vi "FinalizeHWI.vi"(8 "error in (no error)":errorcluster, 10 "Master Device in":refnum<class "Master Device.lvclass">, 11 "Slave_Line in":refnum<class "Slave_Line.lvclass">) -> (0 "error out":errorcluster, 2 "Master Device out":refnum<class "Master Device.lvclass">, 3 "Slave_Line out":refnum<class "Slave_Line.lvclass">)   [LabVIEW 2013, in "Slave_Line.lvclass"]
uses:
  Slave_Line.lvclass
  Master Device/Master Device.lvclass
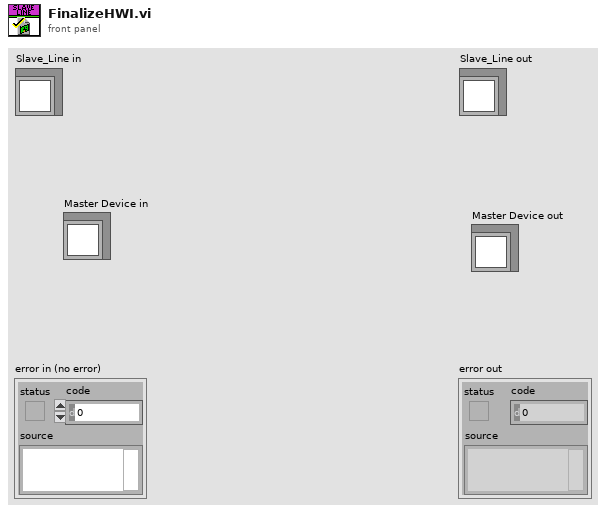
[diagram p1: front panel]
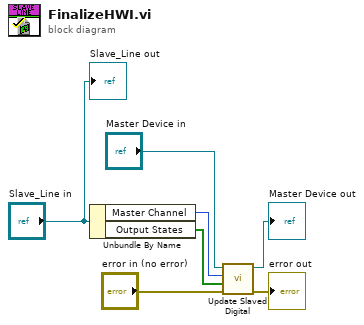
[diagram p0: block diagram]
diagram:
  n1 = Unbundle By Name("Slave_Line in") -> ("Master Channel"=w2:i32, "Output States"=w1:bool[])
  n2 = call-dynamic "Update Slaved Digital.vi"("error in (no error)"="error in (no error)", "Output States"=w1, "Master Channel Number"=w2, "Master Device in"="Master Device in") -> ("error out"=→"error out":errorcluster, "Master Device out"=→"Master Device out":refnum<class "Master Device.lvclass">)  [unwired: 6 in]
  "Slave_Line out" <- "Slave_Line in"
